vi "onDisconnection.vi"(8 "error in (no error)":errorcluster, 11 "Connection.TCP":refnum<class "Connection.TCP.lvclass">) -> (0 "error out":errorcluster, 3 "No Connection":refnum<class "Connection.TCP.lvclass">)   [LabVIEW 2013, in "Connection.TCP_GOSPL.lvlib" / "Connection.TCP.lvclass"]
uses:
  Connection.TCP.lvclass
  Connection/Connection.lvclass
  Connection.TCP.lvclass/Connection.TCP.ctl
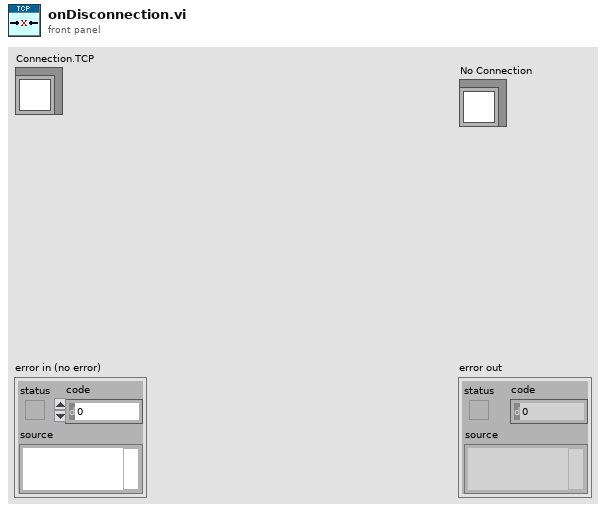
[diagram p1: front panel]
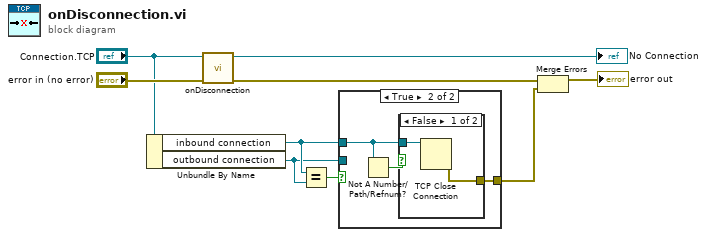
[diagram p0: block diagram]
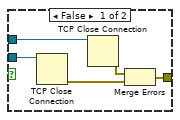
[diagram p2: hidden frame]
diagram:
  n1 = Unbundle By Name("Connection.TCP") -> ("inbound connection"=w4:refnum<k5>, "outbound connection"=w3:refnum<k5>)
  n2 = call-parent "onDisconnection.vi"("error in (no error)"="error in (no error)", "Connection"="Connection.TCP") -> ("error out"=w7:errorcluster, "No connection"=→"No Connection":refnum<class "Connection.TCP.lvclass">)  [unwired: 8 in]
  n3 = Equal?(x=w4, y=w3) -> (x = y?=w1:bool)
  n4 = case shown="True" w1 {
    tunnel: w4 -> [w14 w16]
    tunnel: w3 -> [w13 _]
    tunnel: [w10 w17] -> w2
    frame False {
      n5 = TCP Close Connection(connection ID=w13) -> (error out=w12:errorcluster)  [unwired: 2 in, 1 out]
      n6 = TCP Close Connection(connection ID=w14) -> (error out=w11:errorcluster)  [unwired: 2 in, 1 out]
      n7 = Merge Errors(w11, w12) -> (w10:errorcluster)
    }
    frame True {
      n8 = Not A Number/Path/Refnum?(number/path/refnum=w16) -> (NaN/Path/Refnum?=w15:bool)
      n9 = case shown="False" w15 {
        tunnel: [w19 _] -> w17
        tunnel: w16 -> [w18 _]
        frame False {
          n10 = TCP Close Connection(connection ID=w18) -> (error out=w19:errorcluster)  [unwired: 2 in, 1 out]
        }
        frame True {
        }
      }
    }
  }
  n11 = Merge Errors(w7, w2) -> (→"error out":errorcluster)
